vi "fpga_ARC Filter Impulse Response.vi"(0 "Initial position":u16, 1 "Initial offset":u32, 2 "Number of taps":u16, 3 "filterStepSize[U32.0]":u32 format="%08x", 4 "input valid":bool=TRUE, 6 "ARC Constants":T2={"bufsize"=512, "bufsize-1"=511, "NChan"=8, "NChan-1"=7, "1/2SymPeriods"=10, "Neg1/2SymPeriods"=-10, "polyOrder-1"=4, "maxDec-1"=24}, 7 "ready for output":bool=TRUE) -> (13 "ready for input":bool, 17 "filter info":T1 {"coef [I32.2]" format="%#_6f"}, 18 "output valid":bool)   [LabVIEW 2011, in "NI_EP_Resample_FPGA.lvlib"]
uses:
  <vilib>/addons/Electrical Power/PQ/Resampling/NI_EP_Resample_FPGA.lvlib
  <vilib>/rvi/FXPMathLib/basic elements/FxpAddSub/XNode/nifxpmath_AddSub.xnode
  <vilib>/rvi/FXPMathLib/basic elements/FxpDiscreteDelay/XNode/nifxpmath_DiscreteDelay.xnode
  <vilib>/rvi/FXPMathLib/sim/FxpSim.dll
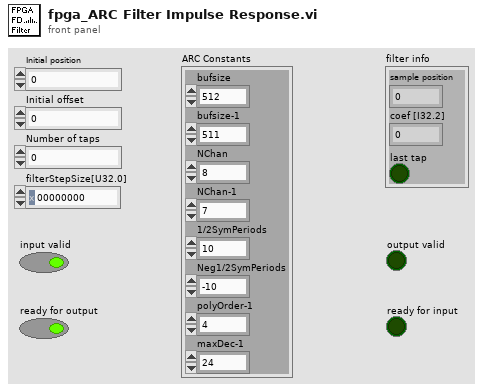
[diagram p1: front panel]
types:
  T1 = cluster{"sample position":u16, "coef [I32.2]":fxp<+/-,32,2>, "last tap":bool}
  T2 = cluster{"bufsize":u16, "bufsize-1":u16, "NChan":u8, "NChan-1":u8, "1/2SymPeriods":i8, "Neg1/2SymPeriods":i8, "polyOrder-1":u8, "maxDec-1":u8}
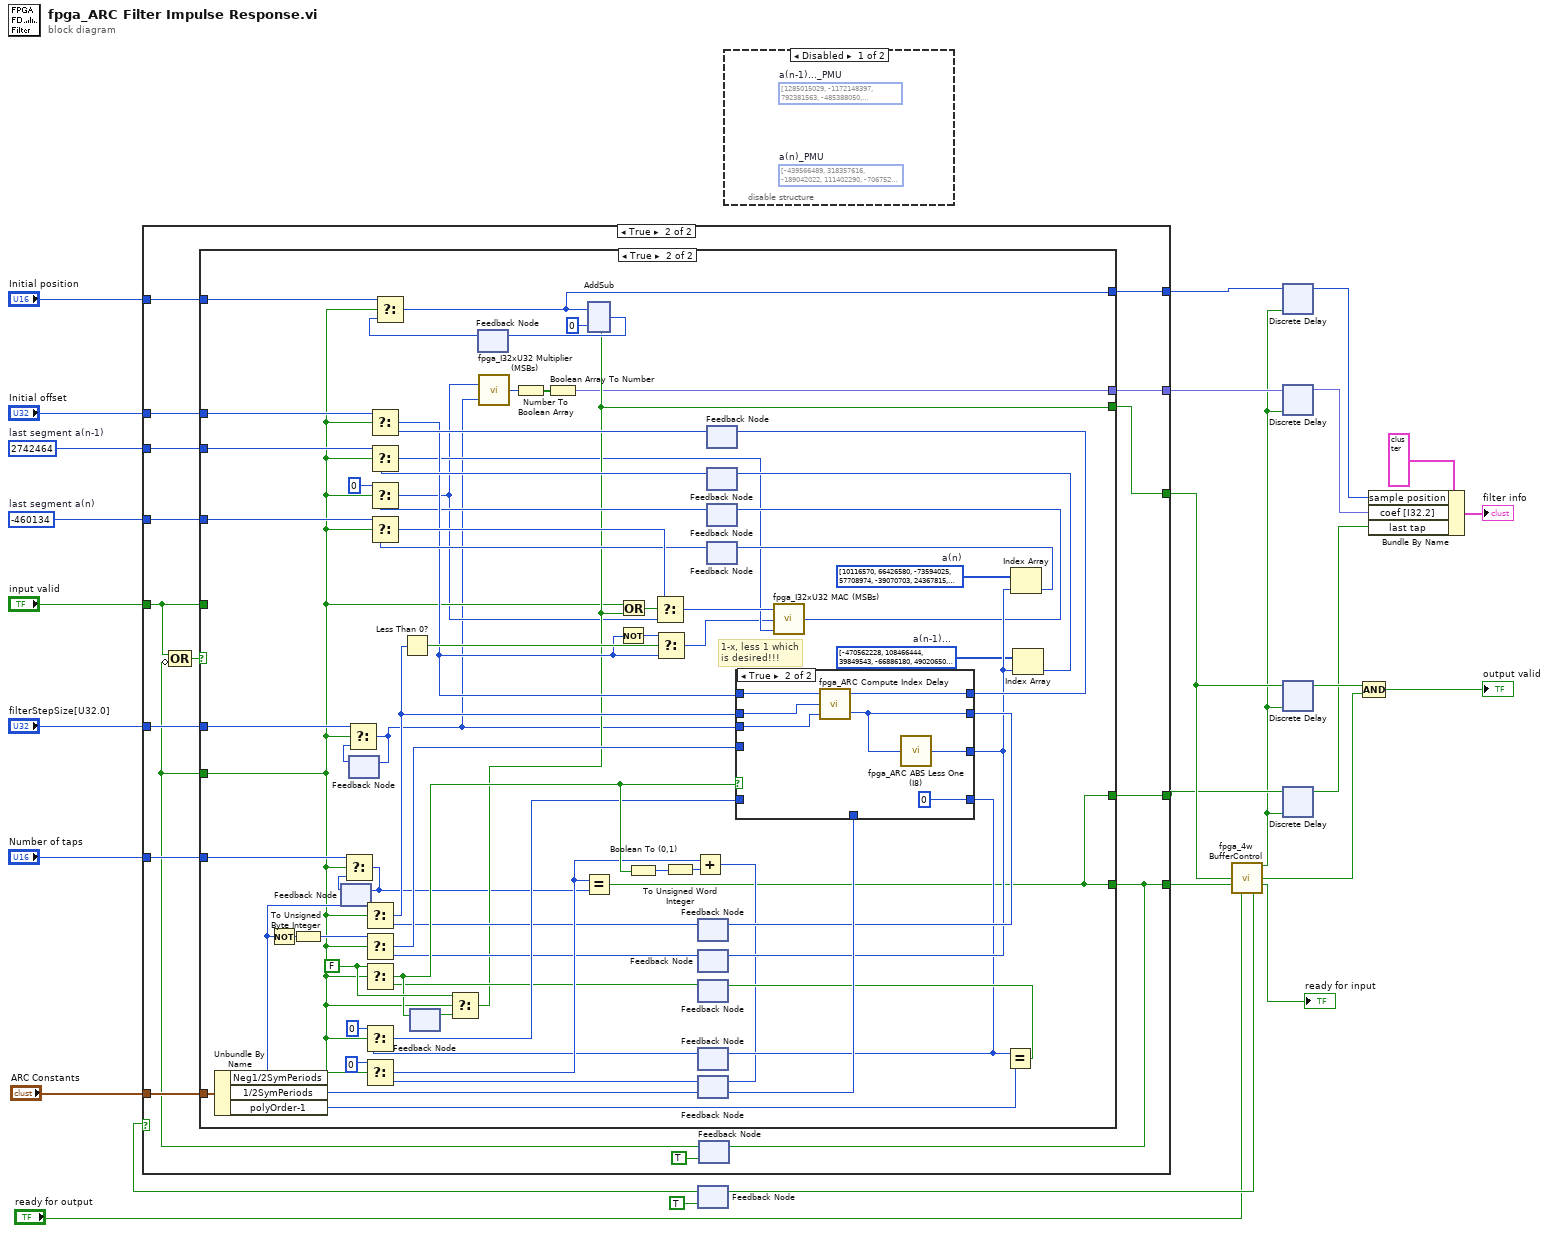
[diagram p0: block diagram]
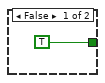
[diagram p4: hidden frame]
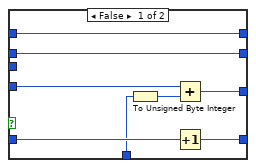
[diagram p5: hidden frame]
diagram:
  w25 = 2742464  # last segment a(n-1)
  w26 = -460134  # last segment a(n)
  n1 = feedback #1(TRUE ("logic enable")) -> (w18:bool)
  n2 = case shown="True" w18 {
    tunnel: "filterStepSize[U32.0]" -> [_ w43]
    tunnel: "Number of taps" -> [_ w42]
    tunnel: "ARC Constants" -> [_ w41]
    tunnel: w26 -> [_ w40]
    tunnel: w25 -> [_ w39]
    tunnel: "Initial offset" -> [_ w38]
    tunnel: [_ w30] -> w8
    tunnel: "input valid" -> [_ w32]
    tunnel: [_ w33] -> w11
    tunnel: [_ w34] -> w12
    tunnel: "Initial position" -> [_ w37]
    tunnel: [_ w35] -> w13
    tunnel: [_ w29] -> w9
    frame False {
    }
    frame True {
      n3 = feedback #2(TRUE) -> (w28:bool)
      n4 = Compound Arithmetic op=OR(w32, invert w28) -> (w36:bool)
      n5 = case shown="True" w36 {
        tunnel: w43 -> [_ w60]
        tunnel: w42 -> [_ w58]
        tunnel: w41 -> [_ w108]
        tunnel: w40 -> [_ w99]
        tunnel: w39 -> [_ w94]
        tunnel: w38 -> [_ w93]
        tunnel: w37 -> [_ w73]
        tunnel: [_ w69] -> w35
        tunnel: [_ w63] -> w33
        tunnel: [_ w51] -> w34
        tunnel: [TRUE w62] -> w30
        tunnel: w32 -> [_ _]
        tunnel: [_ w62] -> w29
        tunnel: w28 -> [_ w56]
        frame False {
        }
        frame True {
          w45 = i32[] [-470562228, 108466444, 39849543, -66886180, 49020650, -27689083, 11616408, -1717216, -3149678, 4578417, -4056058, 2742464, 1324617896, -935174470, 542495163, -297773010, 185939996, -123861555, 83850444, -55786025, 35532498, -21115709, 11317899, -5154777, -182023274, 718704321, -710375257, 459003298, -296675368, 189966390, -118094152, 69884032, -38490791, 19108888, -8067523, 2498024, -1752340362, 1089162759, -285018142, 134513381, -79217883, 51100811, -33874849, 22224304, -14047177, 8345394, -4522133, 2128008, -3629135, -1047585635, 486642718, -286566463, 180003307, -113884377, 70440075, -41675535, 23079935, -11632092, 5093959, -1753585, 1073820532, 0, 0, 0, 0, 0, 0, 0, 0, 0, 0, 0]  # a(n-1)...
          w46 = i32[] [10116570, 66426580, -73594025, 57708974, -39070703, 24367815, -13937926, 7070439, -2924787, 715102, 233856, -460134]  # a(n)
          w83 = FALSE ("t")
          # "1-x, less 1 which\nis desired!!!"
          n6 = Unbundle By Name(w108) -> ("Neg1/2SymPeriods"=w107:i8, "1/2SymPeriods"=w110:i8, "polyOrder-1"=w109:u8)
          n7 = Not(x=w107) -> (.not. x?=w111:i8)
          n8 = To Unsigned Byte Integer(number=w111) -> (unsigned 8bit integer=w106:u8)
          n9 = feedback #3() -> (w59:u16)  [unwired: 1 out]
          n10 = Select(t=w58, s=w56, f=w59) -> (s? t:f=w57:u16)
          n11 = feedback-in #3(w57) -> ()
          n12 = feedback #4() -> (w61:u32)  [unwired: 1 out]
          n13 = Select(t=w60, s=w56, f=w61) -> (s? t:f=w49:u32)
          n14 = feedback-in #4(w49) -> ()
          n15 = feedback #5() -> (w80:bool)  [unwired: 1 out]
          n16 = Select(t=w83, s=w56, f=w80) -> (s? t:f=w63:bool)
          n17 = feedback #6() -> (w70:u16)  [unwired: 1 out]
          n18 = Select(t=w73, s=w56, f=w70) -> (s? t:f=w69:u16)
          n19 = xnode "AddSub"("x"=w69, "y"=u16 0, "carry-in"=w63) -> ("s"=w71:u16)  [unwired: 1 out]
          n20 = feedback-in #6(w71) -> ()
          n21 = Or(x=w56, y=w63) -> (x .or. y?=w103:bool)
          n22 = feedback #7() -> (w67:i8)  [unwired: 1 out]
          n23 = Select(t=w107, s=w56, f=w67) -> (s? t:f=w68:i8)
          n24 = Less Than 0?(x=w68) -> (x < 0?=w104:bool)
          n25 = feedback #8() -> (w66:u8)  [unwired: 1 out]
          n26 = Select(t=w106, s=w56, f=w66) -> (s? t:f=w87:u8)
          n27 = feedback #9() -> (w65:bool)  [unwired: 1 out]
          n28 = Select(t=w83, s=w56, f=w65) -> (s? t:f=w82:bool)
          n29 = feedback-in #5(w82) -> ()
          n30 = Boolean To (0,1)(Boolean=w82) -> (0, 1=w102:i16)
          n31 = To Unsigned Word Integer(number=w102) -> (unsigned 16bit integer=w101:u16)
          n32 = feedback #10() -> (w64:u8)  [unwired: 1 out]
          n33 = Select(t=u8 0, s=w56, f=w64) -> (s? t:f=w77:u8)
          n34 = feedback #11() -> (w76:u16)  [unwired: 1 out]
          n35 = Select(t=u16 0, s=w56, f=w76) -> (s? t:f=w74:u16)
          n36 = Equal?(x=w74, y=w57) -> (x = y?=w62:bool)
          n37 = Add(x=w74, y=w101) -> (x+y=w78:u16)
          n38 = feedback-in #11(w78) -> ()
          n39 = feedback #12() -> (w91:u32)  [unwired: 1 out]
          n40 = Select(t=w93, s=w56, f=w91) -> (s? t:f=w90:u32)
          n41 = Not(x=w90) -> (.not. x?=w105:u32)
          n42 = Select(t=w105, s=w104, f=w90) -> (s? t:f=w52:u32)
          n43 = feedback #13() -> (w96:i32)  [unwired: 1 out]
          n44 = Select(t=w94, s=w56, f=w96) -> (s? t:f=w53:i32)
          n45 = feedback #14() -> (w85:i32)  [unwired: 1 out]
          n46 = Select(t=0, s=w56, f=w85) -> (s? t:f=w50:i32)
          n47 = call <vilib>:"fpga_I32xU32 Multiplier (MSBs).vi"("y[U32]"=w49, "x[I32]"=w50) -> ("x*y[I32 MSB]"=w48:i32)
          n48 = Number To Boolean Array(number=w48) -> (Boolean array=w47:bool[])
          n49 = Boolean Array To Number(Boolean array=w47) -> (number=w51:fxp<+/-,32,2>)
          n50 = feedback #15() -> (w95:i32)  [unwired: 1 out]
          n51 = Select(t=w99, s=w56, f=w95) -> (s? t:f=w98:i32)
          n52 = Select(t=w98, s=w103, f=w50) -> (s? t:f=w55:i32)
          n53 = case shown="True" w82 {
            tunnel: w90 -> [w167 w175]
            tunnel: w68 -> [w168 w174]
            tunnel: w49 -> [_ w173]
            tunnel: [w167 w172] -> w92
            tunnel: [w168 w171] -> w89
            tunnel: w87 -> [w166 _]
            tunnel: [w165 w170] -> w88
            tunnel: w77 -> [w164 _]
            tunnel: [w163 u8 0] -> w81
            tunnel: w110 -> [w161 _]
            frame False {
              n54 = To Unsigned Byte Integer(number=w161) -> (unsigned 8bit integer=w162:u8)
              n55 = Add(x=w166, y=w162) -> (x+y=w165:u8)
              n56 = Increment(x=w164) -> (x+1=w163:u8)
            }
            frame True {
              n57 = call <vilib>:"fpga_ARC Compute Index Delay.vi"("stepSize"=w173, "currSymbolIndex"=w174, "currFractional"=w175) -> ("nextSymbolIndex"=w171:i8, "nextFractionalDelay"=w172:u32)
              n58 = call <vilib>:"fpga_ARC ABS Less One (I8).vi"("x [I8]"=w171) -> ("abs(x)-1"=w170:u8)
            }
          }
          n59 = feedback-in #7(w89) -> ()
          n60 = feedback-in #8(w88) -> ()
          n61 = feedback-in #10(w81) -> ()
          n62 = feedback-in #12(w92) -> ()
          n63 = call <vilib>:"fpga_I32xU32 MAC (MSBs).vi"("sum[I32]"=w53, "y[U32]"=w52, "x[I32]"=w55) -> ("x*y+sum[I32 MSB]"=w54:i32)
          n64 = feedback-in #14(w54) -> ()
          n65 = Equal?(x=w81, y=w109) -> (x = y?=w86:bool)
          n66 = feedback-in #9(w86) -> ()
          n67 = Index Array(array=w46, index=w88) -> (element=w100:i32)
          n68 = feedback-in #15(w100) -> ()
          n69 = Index Array(array=w45, index=w88) -> (element=w97:i32)
          n70 = feedback-in #13(w97) -> ()
        }
      }
      n71 = feedback-in #2(w30) -> ()
    }
  }
  n72 = disable-structure shown="Disabled" {
    frame Disabled {
      (unwired) i32[] [-439566489, 318357616, -189042022, 111402290, -70675255, 45709285, -28871780, 17162952, -9178737, 4037385]  # a(n)_PMU
      (unwired) i32[] [1285015029, -1172148397, 792381563, -485388050, 304580533, -189229383, 112669550, -62132974, 30173504, -11479231, -149575512, 825285244, -815302207, 528794515, -330991784, 198970844, -111892221, 56597738, -23874883, 6578860, -1767357613, 1070327499, -264943056, 119324398, -69076345, 44469528, -29415216, 19028261, -11592418, 6409153, -2295211, -1041821963, 476905722, -274133153, 166162852, -99920275, 57509667, -30655977, 14472534, -5546168, 1073779797, 0, 0, 0, 0, 0, 0, 0, 0, 0]  # a(n-1)..._PMU
    }
    frame Enabled {
    }
  }
  n73 = call <vilib>:"fpga_4w BufferControl.vi"("DR"=w11, "RFI"=w8, "RFO"="ready for output") -> ("buff enable"=w7:bool, "output valid"=w6:bool, "ready for input"=→"ready for input":bool, "logic enable"=w19:bool)  [unwired: 9 in]
  n74 = feedback-in #1(w19) -> ()
  n75 = xnode "Discrete Delay"("D"=w13, "enable"=w7) -> ("Q"=w14:u16)
  n76 = xnode "Discrete Delay"("D"=w12, "enable"=w7) -> ("Q"=w4:fxp<+/-,32,2>)
  n77 = xnode "Discrete Delay"("D"=w11, "enable"=w7) -> ("Q"=w10:bool)
  n78 = xnode "Discrete Delay"("D"=w9, "enable"=w7) -> ("Q"=w3:bool)
  n79 = Compound Arithmetic op=AND(w10, w6) -> (→"output valid":bool)
  n80 = Bundle By Name(cluster=T1 {"sample position"=0, "coef [I32.2]"=0.0, "last tap"=FALSE} ("filter info"), "sample position"=w14, "coef [I32.2]"=w4, "last tap"=w3) -> (→"filter info":T1)
